vi "DIAdem Show Window.vi"(6 "asynchronous? (F)":bool, 7 "bring to front? (F)":bool, 8 "error in (no error)":errorcluster, 9 "mode":T1, 10 "window":T2 items=["SHELL"=0, "NAVIGATOR"=1, "VIEW"=4, "ANALYSIS"=2, "REPORT"=3, "SCRIPT"=7], 11 "DIAdem Reference":T3) -> (0 "error out":errorcluster, 3 "DIAdem Reference":T3)   [LabVIEW 2017]
doc: "Manipulates the display mode of a select component of the DIAdem environment including the whole environment. Several different display modes can be selected.\n\nWhen one of the DIAdem panels is selected, the action (e.g. minimize, maximize) is applied within the DIAdem shell."
uses:
  <vilib>/ExportToExcel/DIAdem Reference.ctl
  <vilib>/ExportToExcel/Window Names.ctl
  <vilib>/ExportToExcel/Window Modes.ctl
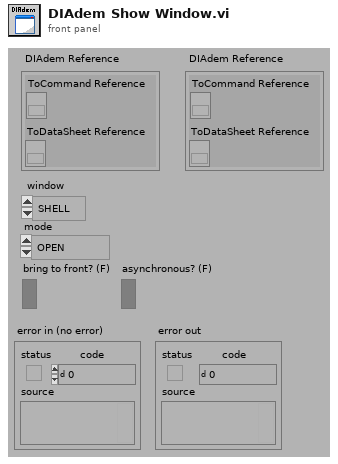
[diagram p1: front panel]
types:
  T1 = typedef "Window Modes.ctl" = enum16{"OPEN", "CLOSE", "SHOW", "MAXIMIZE", "MINIMIZE", "NORMAL", "FULLSIZE"}
  T2 = typedef "Window Names.ctl" = u16
  T3 = typedef "DIAdem Reference.ctl" = cluster{"ToCommand Reference":refnum<k7>, "ToDataSheet Reference":refnum<k7>}
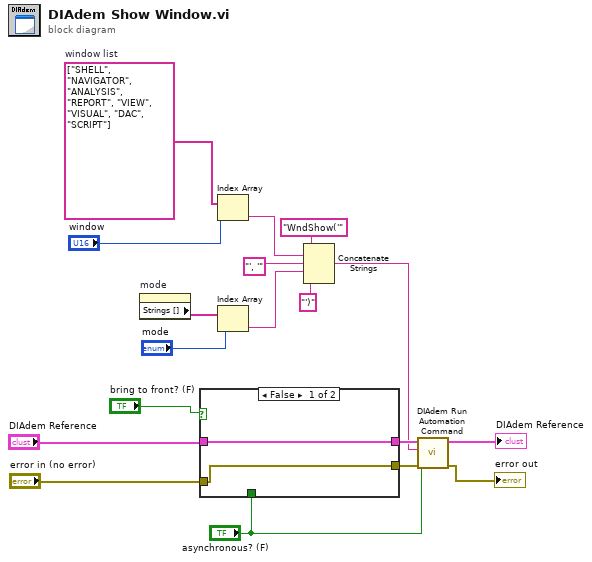
[diagram p0: block diagram]
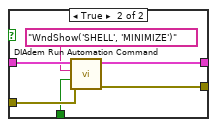
[diagram p2: hidden frame]
diagram:
  w1 = string[] ["SHELL", "NAVIGATOR", "ANALYSIS", "REPORT", "VIEW", "VISUAL", "DAC", "SCRIPT"]  # window list
  n1 = property on="mode" class="Enum (strict)"() -> ("Strings []"=w17:string[])  [unwired: 2 in, 2 out]
  n2 = case shown="False" "bring to front? (F)" {
    tunnel: [w20 w26] -> w10
    tunnel: [w19 w25] -> w9
    tunnel: "error in (no error)" -> [w19 w24]
    tunnel: "DIAdem Reference" -> [w20 w23]
    tunnel: "asynchronous? (F)" -> [_ w22]
    frame False {
    }
    frame True {
      n3 = call <vilib>:"DIAdem Run Automation Command.vi"("error in (no error)"=w24, "asynchronous? (F)"=w22, "command"="WndShow('SHELL', 'MINIMIZE')", "DIAdem Reference"=w23) -> ("error out"=w25:errorcluster, "DIAdem Reference"=w26:T3)  [unwired: 6 in]
    }
  }
  n4 = Index Array(array=w1, index="window") -> (element=w12:string)
  n5 = Index Array(array=w17, index="mode") -> (element=w11:string)
  n6 = Concatenate Strings("WndShow('" ("command"), w12, "', '" ("command"), w11, "')" ("command")) -> (w6:string)
  n7 = call <vilib>:"DIAdem Run Automation Command.vi"("error in (no error)"=w9, "asynchronous? (F)"="asynchronous? (F)", "command"=w6, "DIAdem Reference"=w10) -> ("error out"=→"error out":errorcluster, "DIAdem Reference"=→"DIAdem Reference":T3)  [unwired: 6 in]
